vi "System2.vi"() -> ()   [LabVIEW 2015]
uses:
  <vilib>/DAQmx/write.llb/DAQmx Write (Digital 1D Bool NChan 1Samp 1Line).vi
  <vilib>/DAQmx/write.llb/DAQmx Write (Analog DBL 1Chan 1Samp).vi
  <vilib>/Analysis/baseanly.llb/Mean (DBL).vi
  <vilib>/DAQmx/read.llb/DAQmx Read (Analog 1D DBL 1Chan NSamp).vi
  <vilib>/DAQmx/miscellaneous.llb/DAQmx Fill In Error Info.vi
  <vilib>/addons/control/pid/NI_PID_autopid.lvlib
  <vilib>/Analysis/NI_AALBase.lvlib
panel:
  in  "Open/Close (Green)":bool
  in  "Open/Close (Blue)":bool
  in  "Stop program":bool
  in  "On/Off":bool
  in  "Manual Control 2":bool
  in  "Voltage setting 2":dbl format="%#_13g"
  out "Voltage Reading(pressure) 2":dbl format="%#_13g"
  out "Pressure 2":dbl format="%#.3g"
  out "Pressure Chart 2":dbl(graph)
  in  "autotuning parameters 2":T1={"controller type"=1, "relay cycles"=3, "relay amplitude"=1.0, "control specification"=2, "PV noise level"=0.1} {"PV noise level" format="%.2f"; "control specification" items=["normal", "fast", "slow"]; "relay amplitude" format="%.2f"; "controller type" items=["PID", "PI", "P"]}
  in  "PID gains 2":T2={"proportional gain (Kc)"=1.0, "integral time (Ti, min)"=0.01, "derivative time (Td, min)"=0.0} {"derivative time (Td, min)" format="%.3f"; "integral time (Ti, min)" format="%.3f"; "proportional gain (Kc)" format="%.3f"}
  out "PID gains out 2":T2={"proportional gain (Kc)"=1.0, "integral time (Ti, min)"=0.01, "derivative time (Td, min)"=0.0} {"derivative time (Td, min)" format="%.3f"; "integral time (Ti, min)" format="%.3f"; "proportional gain (Kc)" format="%.3f"}
  in  "autotune? (F) 2":bool
  in  "reinitialize? (F) 2":bool
  in  "setpoint in Bar 2":dbl format="%#.5f"
  out "Control Value 2":dbl
  in  "Voltage setting":dbl format="%#_13g"
  in  "Manual Control":bool
  out "Control Value":dbl
  in  "setpoint in Bar":dbl format="%#.5f"
  in  "reinitialize? (F)":bool
  in  "autotune? (F)":bool
  out "PID gains out":T2={"proportional gain (Kc)"=1.0, "integral time (Ti, min)"=0.01, "derivative time (Td, min)"=0.0} {"derivative time (Td, min)" format="%.3f"; "integral time (Ti, min)" format="%.3f"; "proportional gain (Kc)" format="%.3f"}
  in  "PID gains":T2={"proportional gain (Kc)"=1.0, "integral time (Ti, min)"=0.01, "derivative time (Td, min)"=0.0} {"derivative time (Td, min)" format="%.3f"; "integral time (Ti, min)" format="%.3f"; "proportional gain (Kc)" format="%.3f"}
  in  "autotuning parameters":T1={"controller type"=1, "relay cycles"=3, "relay amplitude"=1.0, "control specification"=2, "PV noise level"=0.1} {"PV noise level" format="%.2f"; "control specification" items=["normal", "fast", "slow"]; "relay amplitude" format="%.2f"; "controller type" items=["PID", "PI", "P"]}
  out "Pressure Chart":dbl(graph)
  out "Pressure":dbl format="%#.3g"
  out "Voltage Reading(pressure)":dbl format="%#_13g"
  # "Pressure Vessel 2"
  # "Pressure Vessel 1"
  # "Readings"
  # "Controls"
  # "Readings"
  # "Controls"
  # "PID Settings"
  # "51.12139\n\n0.044676"
  # "Valves"
  # "Pump 3"
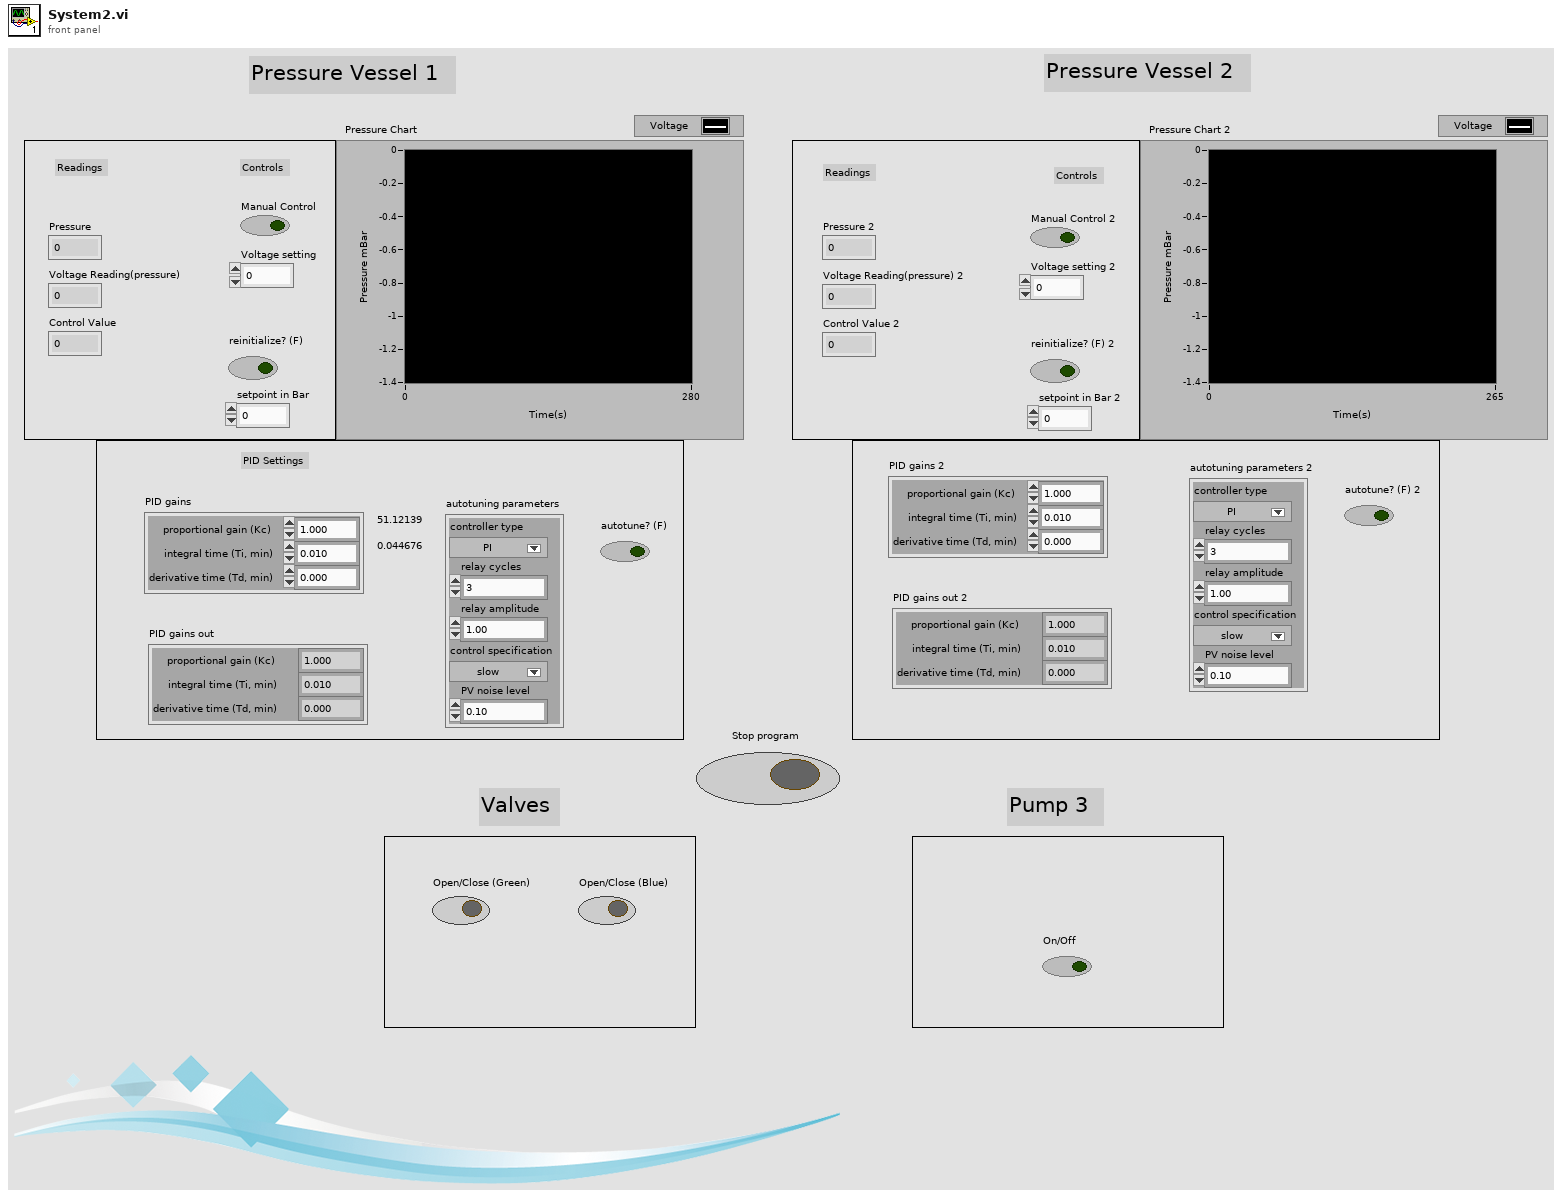
[diagram p1: front panel]
types:
  T1 = cluster{"controller type":u16, "relay cycles":i32, "relay amplitude":dbl, "control specification":u16, "PV noise level":dbl}
  T2 = cluster{"proportional gain (Kc)":dbl, "integral time (Ti, min)":dbl, "derivative time (Td, min)":dbl}
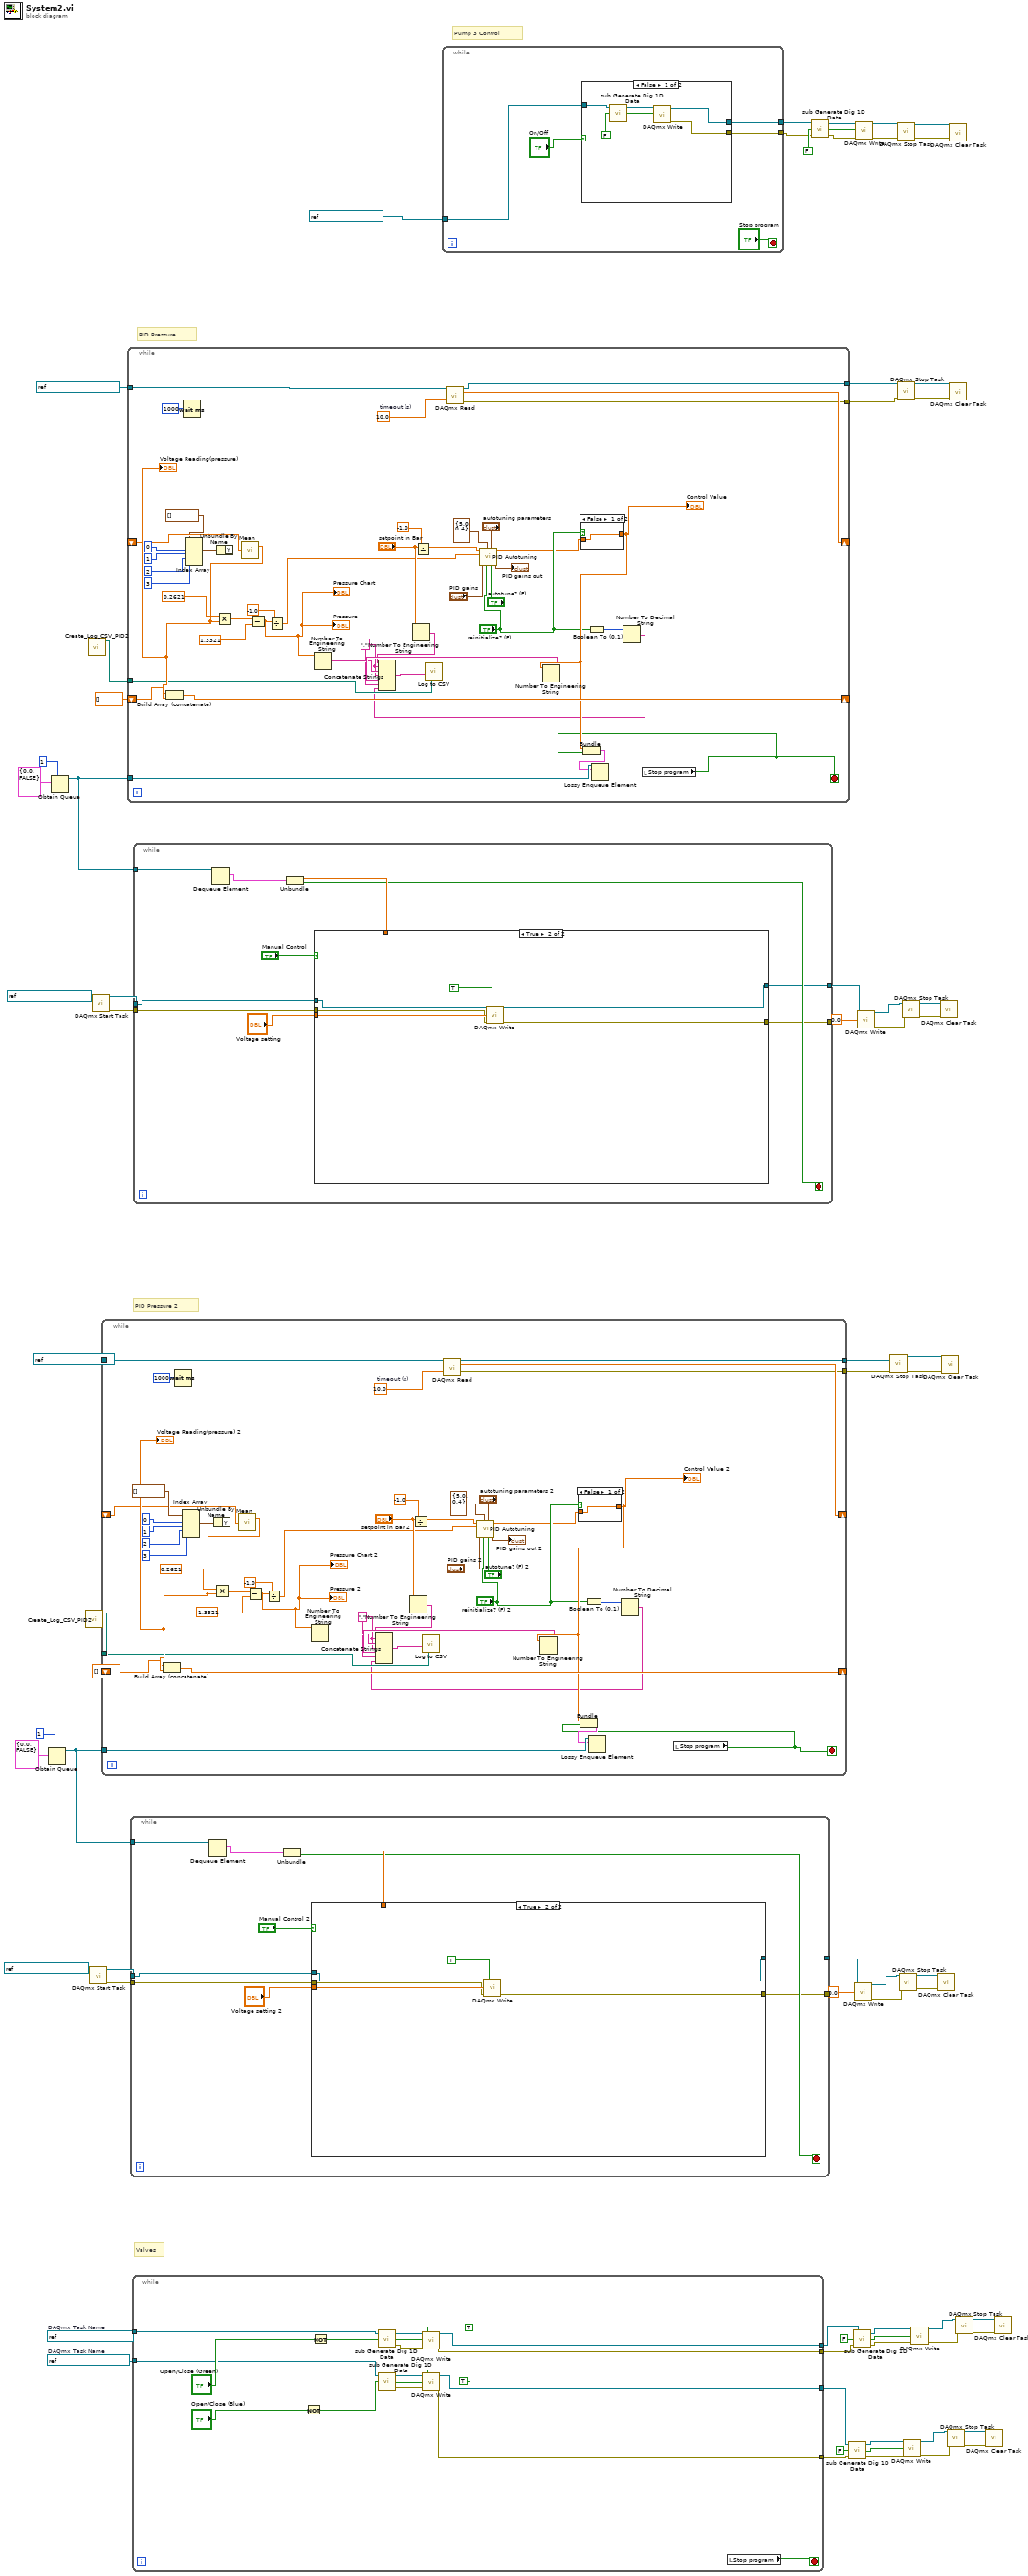
[diagram p0: block diagram]
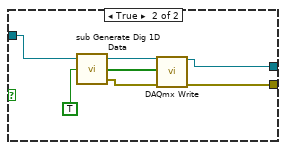
[diagram p2: hidden frame]
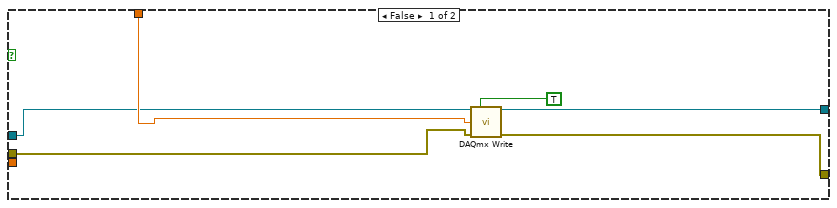
[diagram p3: hidden frame]
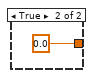
[diagram p4: hidden frame]
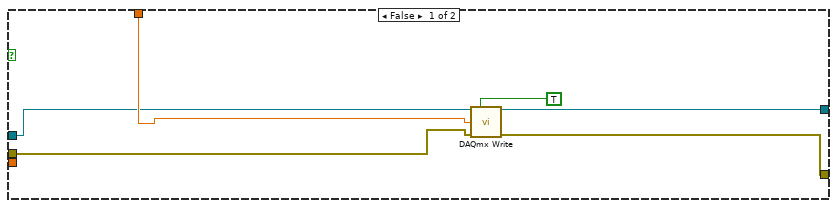
[diagram p5: hidden frame]
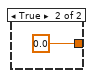
[diagram p6: hidden frame]
diagram:
  w25 = refnum<k21> "NewDigitalSystemBlue"  # DAQmx Task Name
  w26 = refnum<k21> "NewDigitalSystemGreen"  # DAQmx Task Name
  # "Valves"
  # "Pump 3 Control"
  # "PID Pressure"
  # "PID Pressure 2"
  n1 = Obtain Queue(max queue size (-1, unlimited)=1, element data type=cluster{dbl, bool} {0.0, FALSE}) -> (queue out=w54:refnum<queue>)  [unwired: 3 in, 2 out]
  n2 = Obtain Queue(max queue size (-1, unlimited)=1, element data type=cluster{dbl, bool} {0.0, FALSE}) -> (queue out=w69:refnum<queue>)  [unwired: 3 in, 2 out]
  n3 = call "Create_Log_CSV_PID2.vi"() -> ("path"=w50:path)  [unwired: 11 in]
  n4 = call "Create_Log_CSV_PID2.vi"() -> ("path"=w65:path)  [unwired: 11 in]
  n5 = call <vilib>:"DAQmx Start Task.vi"("task/channels in"=refnum<k21> "NewAnalogSystemAO1") -> ("task out"=w49:refnum<k21>, "error out"=w48:errorcluster)  [unwired: 13 in]
  n6 = call <vilib>:"DAQmx Start Task.vi"("task/channels in"=refnum<k21> "NewAnalogSystemAO0") -> ("task out"=w64:refnum<k21>, "error out"=w63:errorcluster)  [unwired: 13 in]
  n7 = while {
    tunnel: refnum<k21> "NewAnalogSystemAI1" -> [w111]
    shift-right: [w105] -> _
    shift-left: _ -> [w72]
    tunnel: w54 -> [w104]
    shift-right: [w96] -> _
    shift-left: dbl[] [] -> [w97]
    tunnel: w50 -> [w90]
    tunnel: [w76] -> w2
    tunnel: [w75] -> w1
    stop <- w77 stop-if-true
    w85 = ","
    w115 = 10.0  # timeout (s)
    n8 = Wait (ms)(milliseconds to wait=u32 1000) -> ()  [unwired: 1 out]
    n9 = Index Array(array=waveform(dbl)[] [] ("data"), index #1=0 ("index"), index #2=1 ("index"), index #3=2 ("index"), index #4=3 ("index")) -> (element #1=w99:waveform(dbl))  [unwired: 3 out]
    n10 = Unbundle By Name(w99) -> ()  [unwired: 1 out]
    n11 = call-poly <vilib>:"Mean.vi"("X"=w72) -> ("mean"=w98:dbl)  [unwired: 1 out]
    "Voltage Reading(pressure) 2" <- w98
    n12 = Build Array (concatenate)(w97, w98) -> (w96:dbl[])
    n13 = Multiply(x=0.2621, y=w98) -> (x*y=w113:dbl)
    n14 = Subtract(x=w113, y=1.3321) -> (x-y=w94:dbl)
    "Pressure 2" <- w94
    "Pressure Chart 2" <- w94
    n15 = Divide(x=w94, y=-1.0) -> (x/y=w82:dbl)
    n16 = Number To Engineering String(4:w94) -> (0:w89:string)  [unwired: 3 in]
    n17 = Number To Engineering String(4:"setpoint in Bar 2") -> (0:w88:string)  [unwired: 3 in]
    n18 = Divide(x="setpoint in Bar 2", y=-1.0) -> (x/y=w81:dbl)
    n19 = call-poly <vilib>:"DAQmx Read.vi"("task/channels in"=w111, "timeout"=w115) -> ("task out"=w76:refnum<k21>, "data"=w105:dbl[], "error out"=w75:errorcluster)  [unwired: 11 in]
    n20 = call <vilib>:"PID Autotuning.vi"("autotune? (F)"="autotune? (F) 2", "autotuning parameters"="autotuning parameters 2", "reinitialize? (F)"="reinitialize? (F) 2", "output range"=cluster{"output high":dbl, "output low":dbl} {"output high"=5.0, "output low"=0.4}, "PID gains"="PID gains 2", "process variable"=w82, "setpoint"=w81) -> ("PID gains out"=→"PID gains out 2":T2, "output"=w79:dbl)  [unwired: 1 in, 2 out]
    n21 = case shown="False" "reinitialize? (F) 2" {
      tunnel: [w116 0.0] -> w93
      tunnel: w79 -> [w116 _]
      frame False {
      }
      frame True {
      }
    }
    "Control Value 2" <- w93
    n22 = Number To Engineering String(4:w93) -> (0:w92:string)  [unwired: 3 in]
    n23 = Boolean To (0,1)(Boolean="reinitialize? (F) 2") -> (0, 1=w86:i16)
    n24 = Number To Decimal String(number=w86) -> (decimal integer string=w84:string)  [unwired: 1 in]
    n25 = Concatenate Strings(w88, w85, w89, w85, w92, w85, w84) -> (w91:string)
    n26 = call "Log to CSV.vi"("Data Str"=w91, "Path"=w90) -> ()  [unwired: 5 in, 1 out]
    n27 = local read "Stop program"() -> (w77:bool)
    n28 = Bundle("output"=w93, "Stop program"=w77) -> (w78:cluster{"output":dbl, "Stop program":bool})  [unwired: 1 in]
    n29 = Lossy Enqueue Element(queue=w104, element=w78) -> ()  [unwired: 1 in, 4 out]
  }
  n30 = while {
    tunnel: refnum<k21> "New AnalogSystemAI0" -> [w157]
    shift-right: [w151] -> _
    shift-left: _ -> [w119]
    tunnel: w69 -> [w150]
    shift-right: [w141] -> _
    shift-left: dbl[] [] -> [w142]
    tunnel: w65 -> [w135]
    tunnel: [w123] -> w28
    tunnel: [w122] -> w27
    stop <- w121 stop-if-true
    w130 = ","
    w161 = 10.0  # timeout (s)
    n31 = Wait (ms)(milliseconds to wait=u32 1000) -> ()  [unwired: 1 out]
    n32 = Index Array(array=waveform(dbl)[] [] ("data"), index #1=0 ("index"), index #2=1 ("index"), index #3=2 ("index"), index #4=3 ("index")) -> (element #1=w144:waveform(dbl))  [unwired: 3 out]
    n33 = Unbundle By Name(w144) -> ()  [unwired: 1 out]
    n34 = call-poly <vilib>:"Mean.vi"("X"=w119) -> ("mean"=w143:dbl)  [unwired: 1 out]
    "Voltage Reading(pressure)" <- w143
    n35 = Build Array (concatenate)(w142, w143) -> (w141:dbl[])
    n36 = Multiply(x=0.2621, y=w143) -> (x*y=w159:dbl)
    n37 = Subtract(x=w159, y=1.3321) -> (x-y=w139:dbl)
    "Pressure" <- w139
    "Pressure Chart" <- w139
    n38 = Divide(x=w139, y=-1.0) -> (x/y=w127:dbl)
    n39 = Number To Engineering String(4:w139) -> (0:w134:string)  [unwired: 3 in]
    n40 = Number To Engineering String(4:"setpoint in Bar") -> (0:w133:string)  [unwired: 3 in]
    n41 = Divide(x="setpoint in Bar", y=-1.0) -> (x/y=w126:dbl)
    n42 = call-poly <vilib>:"DAQmx Read.vi"("task/channels in"=w157, "timeout"=w161) -> ("task out"=w123:refnum<k21>, "data"=w151:dbl[], "error out"=w122:errorcluster)  [unwired: 11 in]
    n43 = call <vilib>:"PID Autotuning.vi"("autotune? (F)"="autotune? (F)", "autotuning parameters"="autotuning parameters", "reinitialize? (F)"="reinitialize? (F)", "output range"=cluster{"output high":dbl, "output low":dbl} {"output high"=5.0, "output low"=0.4}, "PID gains"="PID gains", "process variable"=w127, "setpoint"=w126) -> ("PID gains out"=→"PID gains out":T2, "output"=w124:dbl)  [unwired: 1 in, 2 out]
    n44 = case shown="False" "reinitialize? (F)" {
      tunnel: [w162 0.0] -> w138
      tunnel: w124 -> [w162 _]
      frame False {
      }
      frame True {
      }
    }
    "Control Value" <- w138
    n45 = Number To Engineering String(4:w138) -> (0:w137:string)  [unwired: 3 in]
    n46 = Boolean To (0,1)(Boolean="reinitialize? (F)") -> (0, 1=w131:i16)
    n47 = Number To Decimal String(number=w131) -> (decimal integer string=w129:string)  [unwired: 1 in]
    n48 = Concatenate Strings(w133, w130, w134, w130, w137, w130, w129) -> (w136:string)
    n49 = call "Log to CSV.vi"("Data Str"=w136, "Path"=w135) -> ()  [unwired: 5 in, 1 out]
    n50 = local read "Stop program"() -> (w121:bool)
    n51 = Bundle("output"=w138, "Stop program"=w121) -> (w149:cluster{"output":dbl, "Stop program":bool})  [unwired: 1 in]
    n52 = Lossy Enqueue Element(queue=w150, element=w149) -> ()  [unwired: 1 in, 4 out]
  }
  n53 = while {
    tunnel: w54 -> [w173]
    tunnel: w49 -> [w171]
    tunnel: [w166] -> w46
    tunnel: w48 -> [w165]
    tunnel: [w164] -> _
    stop <- w167 stop-if-true
    n54 = Dequeue Element(queue=w173) -> (element=w170:cluster{dbl, bool})  [unwired: 2 in, 3 out]
    n55 = Unbundle(w170) -> (w169:dbl, w167:bool)
    n56 = case shown="True" "Manual Control 2" {
      tunnel: w171 -> [w177 w184]
      tunnel: w169 -> [w178 _]
      tunnel: "Voltage setting 2" -> [_ w183]
      tunnel: [w176 w182] -> w166
      tunnel: w165 -> [w175 w181]
      tunnel: [w174 w180] -> w164
      frame False {
        n57 = call-poly <vilib>:"DAQmx Write.vi"("task/channels in"=w177, "auto start"=TRUE, "data"=w178, "error in"=w175) -> ("task out"=w176:refnum<k21>, "error out"=w174:errorcluster)  [unwired: 9 in, 1 out]
      }
      frame True {
        n58 = call-poly <vilib>:"DAQmx Write.vi"("task/channels in"=w184, "auto start"=TRUE, "data"=w183, "error in"=w181) -> ("task out"=w182:refnum<k21>, "error out"=w180:errorcluster)  [unwired: 9 in, 1 out]
      }
    }
  }
  n59 = while {
    tunnel: w26 -> [w194]
    tunnel: w25 -> [w193]
    tunnel: [w192] -> w15
    tunnel: [w191] -> w11
    tunnel: [w188] -> w8
    tunnel: [w187] -> w6
    stop <- w186 stop-if-true
    n60 = Not(x="Open/Close (Blue)") -> (.not. x?=w204:bool)
    n61 = Not(x="Open/Close (Green)") -> (.not. x?=w203:bool)
    n62 = call <vilib>:"sub Generate Dig 1D Data.vi"("initial value"=w203, "task in"=w194) -> ("error out"=w190:errorcluster, "Data"=w201:bool[], "task out"=w198:refnum<k21>)  [unwired: 1 in]
    n63 = call <vilib>:"sub Generate Dig 1D Data.vi"("initial value"=w204, "task in"=w193) -> ("error out"=w189:errorcluster, "Data"=w200:bool[], "task out"=w199:refnum<k21>)  [unwired: 1 in]
    n64 = call-poly <vilib>:"DAQmx Write.vi"("task/channels in"=w198, "auto start"=TRUE, "data"=w201, "error in"=w190) -> ("task out"=w192:refnum<k21>, "error out"=w188:errorcluster)  [unwired: 9 in, 1 out]
    n65 = call-poly <vilib>:"DAQmx Write.vi"("task/channels in"=w199, "auto start"=TRUE, "data"=w200, "error in"=w189) -> ("task out"=w191:refnum<k21>, "error out"=w187:errorcluster)  [unwired: 9 in, 1 out]
    n66 = local read "Stop program"() -> (w186:bool)
  }
  n67 = while {
    tunnel: w69 -> [w214]
    tunnel: w64 -> [w212]
    tunnel: [w207] -> w61
    tunnel: w63 -> [w206]
    tunnel: [w205] -> _
    stop <- w208 stop-if-true
    n68 = Dequeue Element(queue=w214) -> (element=w211:cluster{dbl, bool})  [unwired: 2 in, 3 out]
    n69 = Unbundle(w211) -> (w210:dbl, w208:bool)
    n70 = case shown="True" "Manual Control" {
      tunnel: w212 -> [w218 w225]
      tunnel: w210 -> [w219 _]
      tunnel: "Voltage setting" -> [_ w224]
      tunnel: [w217 w223] -> w207
      tunnel: w206 -> [w216 w222]
      tunnel: [w215 w221] -> w205
      frame False {
        n71 = call-poly <vilib>:"DAQmx Write.vi"("task/channels in"=w218, "auto start"=TRUE, "data"=w219, "error in"=w216) -> ("task out"=w217:refnum<k21>, "error out"=w215:errorcluster)  [unwired: 9 in, 1 out]
      }
      frame True {
        n72 = call-poly <vilib>:"DAQmx Write.vi"("task/channels in"=w225, "auto start"=TRUE, "data"=w224, "error in"=w222) -> ("task out"=w223:refnum<k21>, "error out"=w221:errorcluster)  [unwired: 9 in, 1 out]
      }
    }
  }
  n73 = while {
    tunnel: refnum<k21> "NewDigSystemP0L2" -> [w230]
    tunnel: [w229] -> w34
    tunnel: [w228] -> w33
    stop <- "Stop program" stop-if-true
    n74 = case shown="False" "On/Off" {
      tunnel: w230 -> [w237 w241]
      tunnel: [w233 w240] -> w229
      tunnel: [w232 w238] -> w228
      frame False {
        n75 = call <vilib>:"sub Generate Dig 1D Data.vi"("initial value"=FALSE, "task in"=w237) -> ("Data"=w235:bool[], "task out"=w236:refnum<k21>)  [unwired: 1 in, 1 out]
        n76 = call-poly <vilib>:"DAQmx Write.vi"("task/channels in"=w236, "data"=w235) -> ("task out"=w233:refnum<k21>, "error out"=w232:errorcluster)  [unwired: 11 in, 1 out]
      }
      frame True {
        n77 = call <vilib>:"sub Generate Dig 1D Data.vi"("initial value"=TRUE, "task in"=w241) -> ("error out"=w239:errorcluster, "Data"=w243:bool[], "task out"=w242:refnum<k21>)  [unwired: 1 in]
        n78 = call-poly <vilib>:"DAQmx Write.vi"("task/channels in"=w242, "data"=w243, "error in"=w239) -> ("task out"=w240:refnum<k21>, "error out"=w238:errorcluster)  [unwired: 10 in, 1 out]
      }
    }
  }
  n79 = call <vilib>:"sub Generate Dig 1D Data.vi"("error in"=w33, "initial value"=FALSE, "task in"=w34) -> ("error out"=w38:errorcluster, "Data"=w36:bool[], "task out"=w37:refnum<k21>)
  n80 = call <vilib>:"sub Generate Dig 1D Data.vi"("error in"=w6, "initial value"=FALSE, "task in"=w11) -> ("error out"=w5:errorcluster, "Data"=w10:bool[], "task out"=w12:refnum<k21>)
  n81 = call <vilib>:"sub Generate Dig 1D Data.vi"("error in"=w8, "initial value"=FALSE, "task in"=w15) -> ("error out"=w7:errorcluster, "Data"=w9:bool[], "task out"=w16:refnum<k21>)
  n82 = call-poly <vilib>:"DAQmx Write.vi"("task/channels in"=w46, "data"=0.0) -> ("task out"=w45:refnum<k21>, "error out"=w44:errorcluster)  [unwired: 11 in, 1 out]
  n83 = call-poly <vilib>:"DAQmx Write.vi"("task/channels in"=w37, "data"=w36, "error in"=w38) -> ("task out"=w32:refnum<k21>, "error out"=w31:errorcluster)  [unwired: 10 in, 1 out]
  n84 = call-poly <vilib>:"DAQmx Write.vi"("task/channels in"=w61, "data"=0.0) -> ("task out"=w60:refnum<k21>, "error out"=w59:errorcluster)  [unwired: 11 in, 1 out]
  n85 = call <vilib>:"DAQmx Stop Task.vi"("task/channels in"=w2, "error in"=w1) -> ("task out"=w3:refnum<k21>, "error out"=w4:errorcluster)  [unwired: 12 in]
  n86 = call <vilib>:"DAQmx Stop Task.vi"("task/channels in"=w32, "error in"=w31) -> ("task out"=w40:refnum<k21>, "error out"=w39:errorcluster)  [unwired: 12 in]
  n87 = call <vilib>:"DAQmx Stop Task.vi"("task/channels in"=w28, "error in"=w27) -> ("task out"=w29:refnum<k21>, "error out"=w30:errorcluster)  [unwired: 12 in]
  n88 = call <vilib>:"DAQmx Stop Task.vi"("task/channels in"=w45, "error in"=w44) -> ("task out"=w47:refnum<k21>, "error out"=w43:errorcluster)  [unwired: 12 in]
  n89 = call <vilib>:"DAQmx Stop Task.vi"("task/channels in"=w60, "error in"=w59) -> ("task out"=w62:refnum<k21>, "error out"=w58:errorcluster)  [unwired: 12 in]
  n90 = call-poly <vilib>:"DAQmx Write.vi"("task/channels in"=w12, "data"=w10, "error in"=w5) -> ("task out"=w19:refnum<k21>, "error out"=w18:errorcluster)  [unwired: 10 in, 1 out]
  n91 = call-poly <vilib>:"DAQmx Write.vi"("task/channels in"=w16, "data"=w9, "error in"=w7) -> ("task out"=w22:refnum<k21>, "error out"=w23:errorcluster)  [unwired: 10 in, 1 out]
  n92 = call <vilib>:"DAQmx Clear Task.vi"("task in"=w47, "error in"=w43) -> ()  [unwired: 13 in, 1 out]
  n93 = call <vilib>:"DAQmx Clear Task.vi"("task in"=w62, "error in"=w58) -> ()  [unwired: 13 in, 1 out]
  n94 = call <vilib>:"DAQmx Clear Task.vi"("task in"=w3, "error in"=w4) -> ()  [unwired: 13 in, 1 out]
  n95 = call <vilib>:"DAQmx Stop Task.vi"("task/channels in"=w19, "error in"=w18) -> ("task out"=w20:refnum<k21>, "error out"=w17:errorcluster)  [unwired: 12 in]
  n96 = call <vilib>:"DAQmx Clear Task.vi"("task in"=w40, "error in"=w39) -> ()  [unwired: 13 in, 1 out]
  n97 = call <vilib>:"DAQmx Clear Task.vi"("task in"=w29, "error in"=w30) -> ()  [unwired: 13 in, 1 out]
  n98 = call <vilib>:"DAQmx Stop Task.vi"("task/channels in"=w22, "error in"=w23) -> ("task out"=w21:refnum<k21>, "error out"=w24:errorcluster)  [unwired: 12 in]
  n99 = call <vilib>:"DAQmx Clear Task.vi"("task in"=w20, "error in"=w17) -> ()  [unwired: 13 in, 1 out]
  n100 = call <vilib>:"DAQmx Clear Task.vi"("task in"=w21, "error in"=w24) -> ()  [unwired: 13 in, 1 out]
